vi "InitDrv.vi"   [LabVIEW 2015]
uses:
  ESLSCDLL.dll
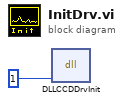
[diagram p0: block diagram]
diagram:
  n1 = dll-call lib="C:/GIT_Repositories/lv64/1cam/board.vis/ESLSCDLL.dll" fn="DLLCCDDrvInit"("drv"=u32 1) -> ()  [unwired: 5 in, 2 out]
